vi "UDP Tx Init.vi"(0 "parameter":T1={"remote IP Address"="192.168.1.101", "remote port"=54322, "local port(Tx)"=54321, "local port(Rx)"=54323}) -> (1 "parameter out":T1={"remote IP Address"="192.168.1.101", "remote port"=54322, "local port(Tx)"=54321, "local port(Rx)"=54323}, 2 "Tx ID":refnum<k16>, 3 "Rx ID":refnum<k16>, 4 "error out":errorcluster)   [LabVIEW 2014]
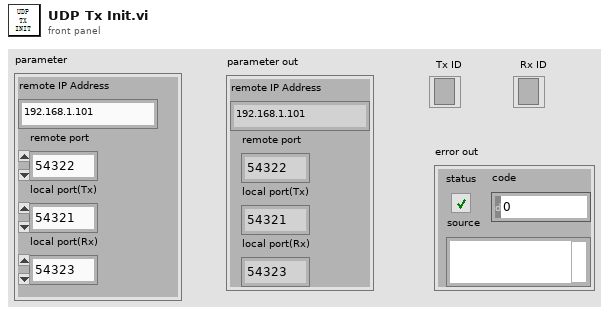
[diagram p1: front panel]
types:
  T1 = cluster{"remote IP Address":string, "remote port":u16, "local port(Tx)":u16, "local port(Rx)":u16}
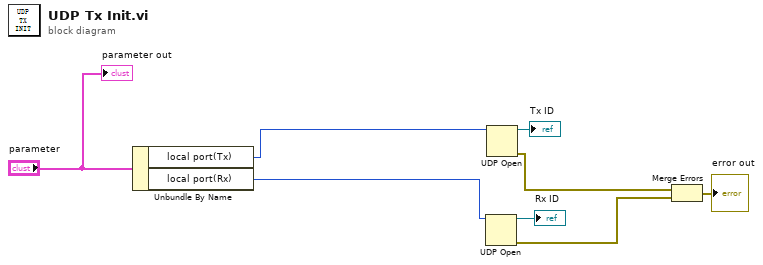
[diagram p0: block diagram]
diagram:
  n1 = Unbundle By Name("parameter") -> ("local port(Tx)"=w7:u16, "local port(Rx)"=w6:u16)
  n2 = UDP Open(11:w6) -> (port=→"Rx ID":refnum<k16>, 0:w2:errorcluster)  [unwired: 4 in, 1 out]
  n3 = UDP Open(11:w7) -> (port=→"Tx ID":refnum<k16>, 0:w3:errorcluster)  [unwired: 4 in, 1 out]
  n4 = Merge Errors(w3, w2) -> (→"error out":errorcluster)
  "parameter out" <- "parameter"
